vi "CPU_Waterfall.vi"(7 "Config":cluster{"History":i32, "X Resolution":i32}={"History"=100, "X Resolution"=400000}, 11 "Spectrum":dbl[](array[numeric]) format="%.2f") -> (1 "DownSampled Waterfall":i16[][](array[numeric]), 3 "DownSampled Spectrum":sgl[](array[numeric]) format="%.2f")   [LabVIEW 2020]
uses:
  <vilib>/Analysis/2dsp.llb/Decimate (single shot, DBL).vi
  <vilib>/Analysis/NI_AALPro.lvlib
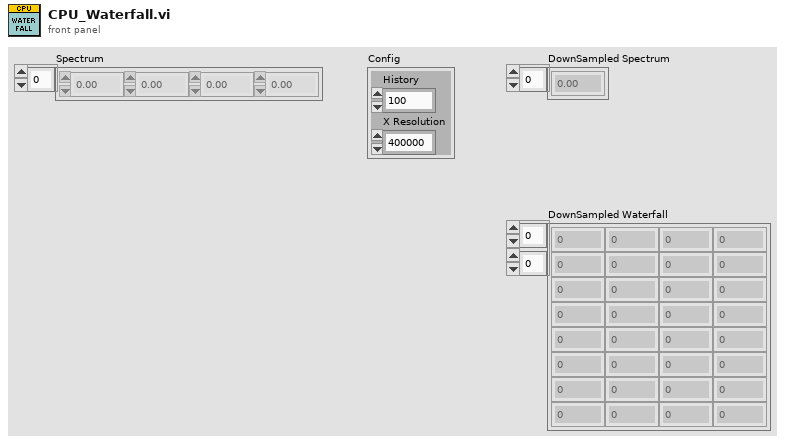
[diagram p1: front panel]
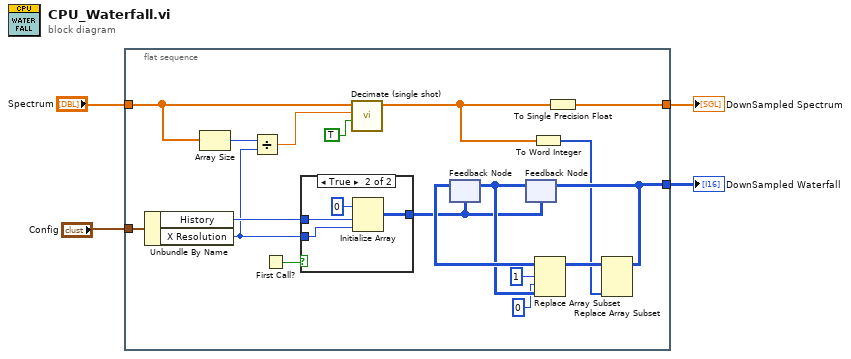
[diagram p0: block diagram]
diagram:
  n1 = flat-sequence {
    tunnel: "Spectrum" -> [w18]
    tunnel: "Config" -> [w20]
    tunnel: [w13] -> w2
    tunnel: [w5] -> w1
    frame #0 {
      n2 = Unbundle By Name(w20) -> ("History"=w17:i32, "X Resolution"=w9:i32)
      n3 = Array Size(array=w18) -> (size(s)=w10:i32)
      n4 = Divide(x=w10, y=w9) -> (x/y=w8:dbl)
      n5 = First Call?() -> (First Call?: T/F=w19:bool)
      n6 = case shown="True" w19 {
        tunnel: [_ w23] -> w11
        tunnel: w17 -> [_ w25]
        tunnel: w9 -> [_ w24]
        frame False {
        }
        frame True {
          n7 = Initialize Array(i16 0 ("element"), w25, w24) -> (w23:i16[][])
        }
      }
      n8 = call-poly <vilib>:"Decimate (single shot).vi"("averaging"=TRUE, "decimating factor"=w8, "X"=w18) -> ("Decimated Array"=w6:dbl[])  [unwired: 7 in, 1 out]
      n9 = feedback #1(w11) -> (w22:i16[][])
      n10 = feedback #2(w11) -> (w21:i16[][])
      n11 = feedback-in #1(w21) -> ()
      n12 = To Word Integer(number=w6) -> (16bit integer=w7:i16[])
      n13 = Replace Array Subset(array=w22, new element=w21, index (row)=1, index (col)=0 ("disabled index (col)")) -> (w14:i16[][])
      n14 = To Single Precision Float(number=w6) -> (single precision float=w5:sgl[])
      n15 = Replace Array Subset(array=w14, new element=w7) -> (w13:i16[][])  [unwired: 2 in]
      n16 = feedback-in #2(w13) -> ()
    }
  }
  "DownSampled Waterfall" <- w2
  "DownSampled Spectrum" <- w1
